vi "PDA_Blast_Acquisition.vi"(4 "Shutter Mode":bool, 5 "Number of Accumulations":i16=5, 6 "error in":errorcluster, 7 "StartIng Mode":T1(ring), 9 "Acquisition Parameters":T2={"Exposure (ms)"=100, "Interval (ms)"=100, "Flush Count"=1, "Trigger"=0} {"Trigger" items=["Disable", "Acquistion", "Cycle"]}) -> (0 "error out":errorcluster, 1 "Pixel Overflow":i32, 2 "PDA Overflow":bool, 3 "Final Data Array":dbl[](array[numeric]) format="%.2f")   [LabVIEW 2019]
doc: "This VI demonstrates acquisition and image display of CCD data\nutilizing the ISA CCD driver.\n\nNote: Specific help is available for each individual control, display and indicator."
uses:
  Globals and TypeDefs/Type Definitions.llb/3 way Status.ctl
  <vilib>/Analysis/baseanly.llb/Mean (DBL).vi
  Globals and TypeDefs/gStatus.vi
  IGA_comm.llb/Controller Version Number.vi
  <vilib>/Analysis/NI_AALBase.lvlib
panel:
  out "Blasttime":u32
  out "Current Mode":T1(ring)
  in  "Tab Control":enum32{"All Accumulations", "Averaged Signal"}(tab)
  out "Display":sgl[][](graph)
  out "Averaged Signal":dbl[](graph)
  out "Avg value":dbl format="%0.2f"
  out "Avg Deviation":dbl format="%0.2f"
  out "Time Used":u32[](array[numeric])
  in  "CCD ADC and Gain":dbl(ring) items=["16 bits Gain 1", "16 bits Gain 2", "16 bits Gain 3", "16 bits Gain 4", "14 bits Gain 1", "14 bits Gain 2"]
  out "Data":u16[][](array[numeric])
  in  "Number of Region":u32=1 min=1 max=1
  # "Total"
  # "Init"
  # "Reset"
  # "SetAcqPara"
  # "SetArea"
  # "Acquisition"
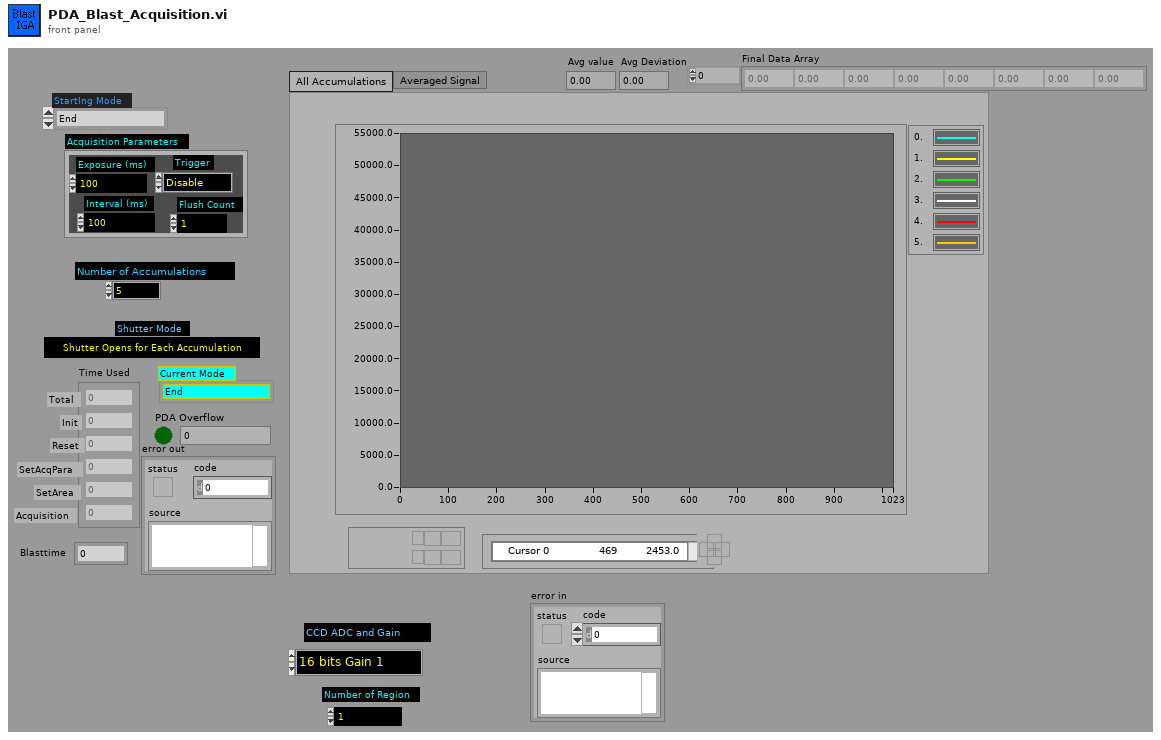
[diagram p1: front panel]
types:
  T1 = enum16{"End", "Init", "Reset", "SetAcqParameter", "SetArea", "AcqData"}
  T2 = cluster{"Exposure (ms)":u32, "Interval (ms)":u32, "Flush Count":i32, "Trigger":u16}
  T3 = typedef "3 way Status.ctl" = u8
  T4 = cluster{"Comm Interface":u16, "BUS":i16, "Address":i16, "Com Port":i32}
  T5 = cluster{"Exposure (ms)":bool, "Interval (ms)":bool, "Flush Count":bool, "Trigger":bool}
  T6 = cluster{"X Origin":u32, "Y Origin":u32, "X Size":u32, "Y Size":u32, "X Bin":u32, "Y Bin":u32}[]
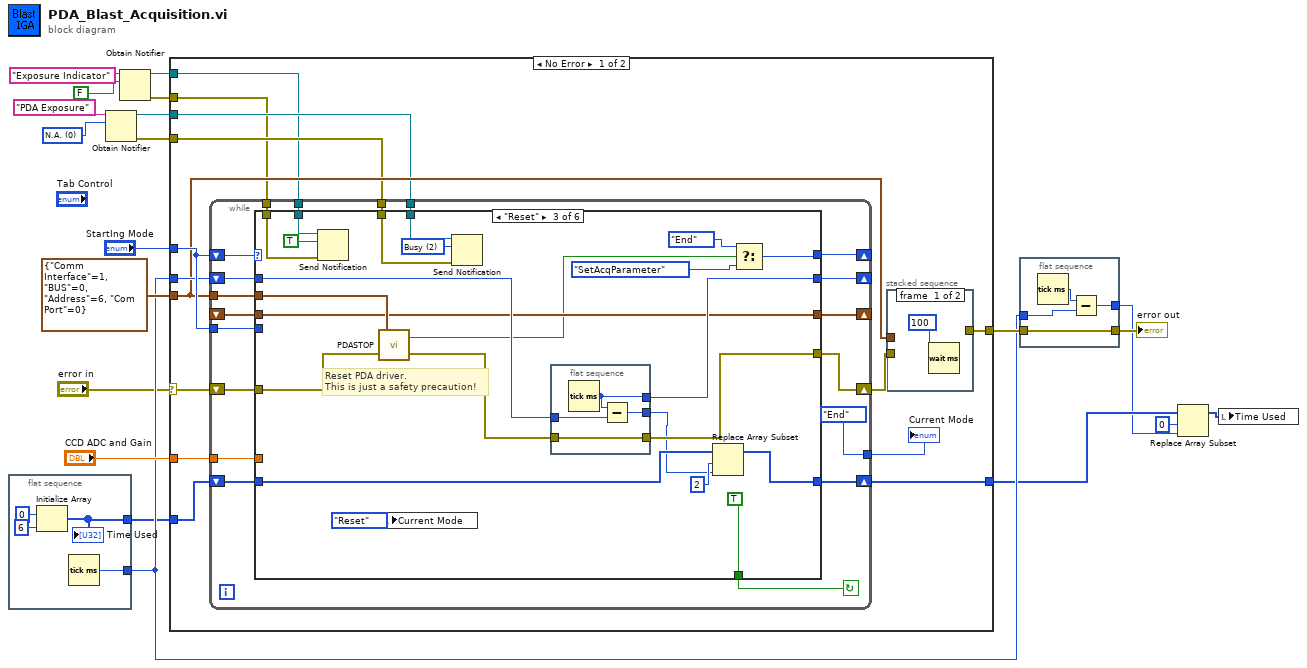
[diagram p0: block diagram]
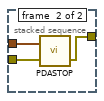
[diagram p2: hidden frame]
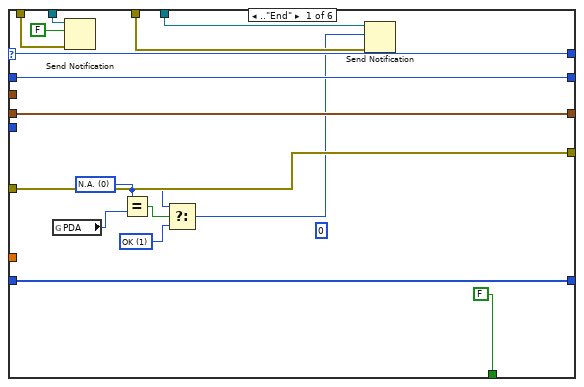
[diagram p3: hidden frame]
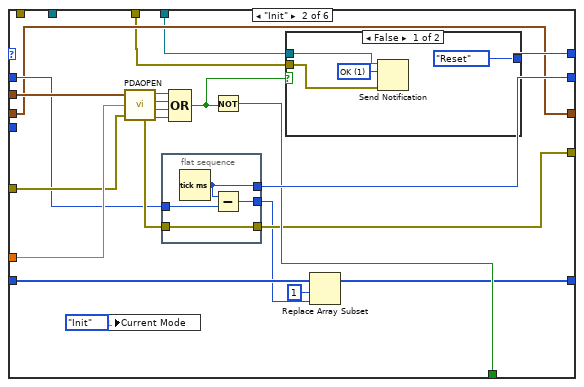
[diagram p4: hidden frame]
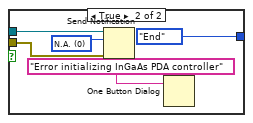
[diagram p5: hidden frame]
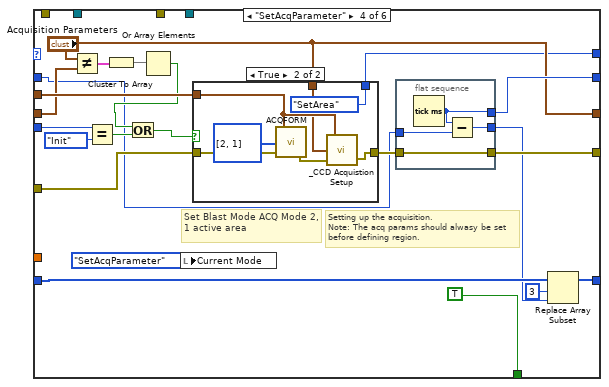
[diagram p6: hidden frame]
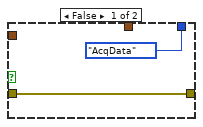
[diagram p7: hidden frame]
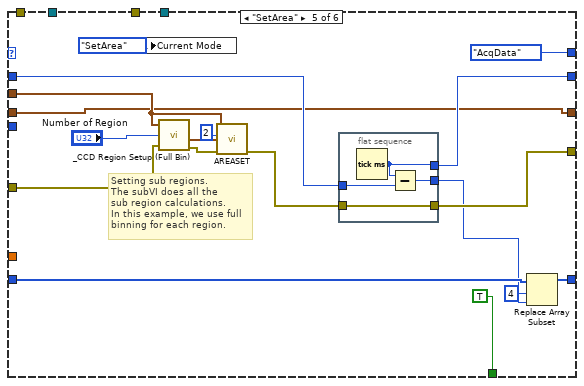
[diagram p8: hidden frame]
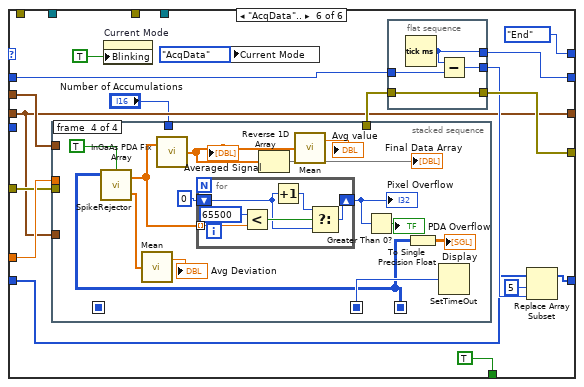
[diagram p9: hidden frame]
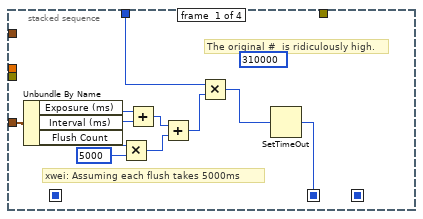
[diagram p10: hidden frame]
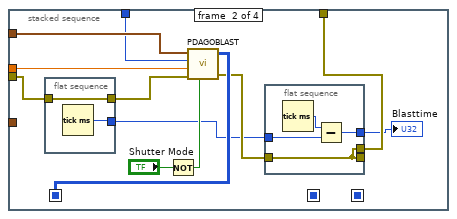
[diagram p11: hidden frame]
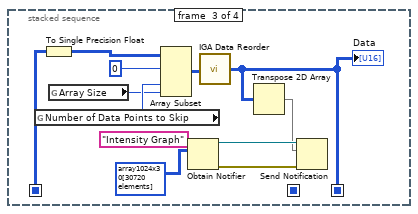
[diagram p12: hidden frame]
diagram:
  w8 = T3 0 items=["N.A.", "OK", "Busy", "Done"] ("Saving")
  n1 = flat-sequence {
    tunnel: [w24] -> w15
    tunnel: [w21] -> w14
    frame #0 {
      n2 = Initialize Array(u32 0 ("element"), 6 ("dimension size")) -> (w21:u32[])
      "Time Used" <- w21
      n3 = Tick Count (ms)() -> (millisecond timer value=w24:u32)
    }
  }
  n4 = Obtain Notifier(name (unnamed)="PDA Exposure", notification data type=w8) -> (notifier out=w7:refnum<notifier>, error out=w6:errorcluster)  [unwired: 2 in, 1 out]
  n5 = Obtain Notifier(name (unnamed)="Exposure Indicator", notification data type=FALSE ("SaveData?")) -> (notifier out=w3:refnum<notifier>, error out=w2:errorcluster)  [unwired: 2 in, 1 out]
  n6 = case shown="No Error" "error in" {
    selector: "error in" -> [w29 w277]
    tunnel: [w38 w277] -> w17
    tunnel: w15 -> [w34 _]
    tunnel: "StartIng Mode" -> [w36 _]
    tunnel: T4 {"Comm Interface"=1, "BUS"=0, "Address"=6, "Com Port"=0} ("Comm Params") -> [w33 _]
    tunnel: "CCD ADC and Gain" -> [w35 _]
    tunnel: w14 -> [w32 w278]
    tunnel: [w31 w278] -> w12
    tunnel: w7 -> [w28 _]
    tunnel: w6 -> [w27 _]
    tunnel: w3 -> [w26 _]
    tunnel: w2 -> [w25 _]
    frame No Error {
      n7 = while {
        tunnel: w35 -> [w57]
        shift-left: _ -> [w58]
        shift-right: [w59] -> _
        shift-left: w36 -> [w51]
        shift-right: [w60] -> _
        shift-right: [w53] -> w37
        shift-left: w29 -> [w56]
        shift-right: [w54] -> _
        shift-left: w34 -> [w55]
        tunnel: w33 -> [w52]
        tunnel: w36 -> [w50]
        shift-right: [w48] -> w31
        shift-left: w32 -> [w49]
        tunnel: [T1."End" ("Current Mode")] -> w30
        tunnel: w28 -> [w46]
        tunnel: w27 -> [w45]
        tunnel: w26 -> [w44]
        tunnel: w25 -> [w43]
        stop <- w61 continue-if-true
        n8 = case shown="\"Reset\"" w51 {
          selector: w51 -> [w76 _ _ _ _ _]
          tunnel: [FALSE w89 TRUE TRUE TRUE TRUE] -> w61
          tunnel: [w76 w86 w121 w145 T1."AcqData" ("InGaAsSS") T1."End" ("InGaAsSS")] -> w60
          tunnel: w58 -> [w75 w85 w128 w155 w182 w199]
          tunnel: [w75 w85 w128 "Acquisition Parameters" w182 w199] -> w59
          tunnel: w57 -> [_ w94 _ _ _ w212]
          tunnel: w56 -> [w73 w93 w134 w160 w176 w211]
          tunnel: w55 -> [w74 w91 w132 w146 w185 w197]
          tunnel: [w74 w90 w131 w157 w186 w208] -> w54
          tunnel: [w73 w88 w130 w158 w187 w209] -> w53
          tunnel: w52 -> [_ w95 w129 w156 w184 w207]
          tunnel: w50 -> [_ _ _ w151 _ _]
          tunnel: w49 -> [w72 w84 w125 w143 w179 w203]
          tunnel: [w72 w81 w126 w142 w180 w202] -> w48
          tunnel: w46 -> [w68 w79 w118 _ _ _]
          tunnel: w45 -> [w67 w78 w117 _ _ _]
          tunnel: w44 -> [w64 _ w115 _ _ _]
          tunnel: w43 -> [w63 _ w114 _ _ _]
          frame .."End" {
            w69 = T3 0 items=["N.A.", "OK", "Busy", "Done"] ("x")
            w65 = T3 1 items=["N.A.", "OK", "Busy", "Done"] ("Saving")
            (unwired) u32 0 ("Read count")
            n9 = global read "gStatus.vi" "PDA"() -> (w71:T3)
            n10 = Send Notification(notification=FALSE, notifier=w64, error in (no error)=w63) -> ()  [unwired: 2 out]
            n11 = Equal?(x=w69, y=w71) -> (x = y?=w70:bool)
            n12 = Select(t=w69, s=w70, f=w65) -> (s? t:f=w66:T3)
            n13 = Send Notification(notification=w66, notifier=w68, error in (no error)=w67) -> ()  [unwired: 2 out]
          }
          frame "Init" {
            n14 = local write "Current Mode"(T1."Init" ("Current Mode")) -> ()
            n15 = call "PDAOPEN.VI"("error in"=w93, "CCD ADC and Gain"=w94, "Comm Params"=w95) -> ("State Error"=w96:bool, "error out"=w92:errorcluster, "Table Error"=w97:bool, "Init Error"=w98:bool, "Boot Error"=w99:bool)  [unwired: 1 out]
            n16 = flat-sequence {
              tunnel: w92 -> [w112]
              tunnel: [w112] -> w88
              tunnel: w91 -> [w111]
              tunnel: [w110] -> w83
              tunnel: [w109] -> w90
              frame #0 {
                n17 = Tick Count (ms)() -> (millisecond timer value=w109:u32)
                n18 = Subtract(x=w109, y=w111) -> (x-y=w110:u32)
              }
            }
            n19 = Compound Arithmetic op=OR(w99, w98, w97, w96) -> (w87:bool)
            n20 = Not(x=w87) -> (.not. x?=w89:bool)
            n21 = case shown="False" w87 {
              tunnel: [T1."Reset" ("InGaAsSS") T1."End" ("InGaAsSS")] -> w86
              tunnel: w79 -> [w102 w106]
              tunnel: w78 -> [w101 w105]
              frame False {
                w100 = T3 1 items=["N.A.", "OK", "Busy", "Done"] ("notification")
                n22 = Send Notification(notification=w100, notifier=w102, error in (no error)=w101) -> ()  [unwired: 2 out]
              }
              frame True {
                w104 = T3 0 items=["N.A.", "OK", "Busy", "Done"] ("notification")
                n23 = Send Notification(notification=w104, notifier=w106, error in (no error)=w105) -> ()  [unwired: 2 out]
                n24 = One Button Dialog(message="Error initializing InGaAs PDA controller") -> ()  [unwired: 1 in, 1 out]
              }
            }
            n25 = Replace Array Subset(array=w84, new element=w83, index=1) -> (w81:u32[])
          }
          frame "Reset" {
            w116 = T3 2 items=["N.A.", "OK", "Busy", "Done"] ("notification")
            # "Reset PDA driver.\nThis is just a safety precaution!"
            n26 = Send Notification(notification=TRUE, notifier=w115, error in (no error)=w114) -> ()  [unwired: 2 out]
            n27 = call "PDASTOP.VI"("error in"=w134, "Comm Params"=w129) -> ("error out"=w133:errorcluster, "Error"=w122:bool)
            n28 = local write "Current Mode"(T1."Reset" ("Current Mode")) -> ()
            n29 = Send Notification(notification=w116, notifier=w118, error in (no error)=w117) -> ()  [unwired: 2 out]
            n30 = flat-sequence {
              tunnel: w133 -> [w139]
              tunnel: [w139] -> w130
              tunnel: w132 -> [w138]
              tunnel: [w137] -> w124
              tunnel: [w136] -> w131
              frame #0 {
                n31 = Tick Count (ms)() -> (millisecond timer value=w136:u32)
                n32 = Subtract(x=w136, y=w138) -> (x-y=w137:u32)
              }
            }
            n33 = Replace Array Subset(array=w125, new element=w124, index=2) -> (w126:u32[])
            n34 = Select(t=T1."End" ("InGaAsSS"), s=w122, f=T1."SetAcqParameter" ("InGaAsSS")) -> (s? t:f=w121:T1)
          }
          frame "SetAcqParameter" {
            # "Setting up the acquisition.\nNote: The acq params should alwasy be set\nbefore defining region."
            # "Set Blast Mode ACQ Mode 2, 1 active area"
            n35 = Not Equal?(x="Acquisition Parameters", y=w155) -> (x != y?=w152:T5)
            n36 = Equal?(x=w151, y=T1."Init") -> (x = y?=w149:bool)
            n37 = Cluster To Array(cluster=w152) -> (array=w153:bool[])
            n38 = Or Array Elements(Boolean array=w153) -> (logical OR=w148:bool)
            n39 = Or(x=w148, y=w149) -> (x .or. y?=w147:bool)
            n40 = local write "Current Mode"(T1."SetAcqParameter" ("Current Mode")) -> ()
            n41 = case shown="True" w147 {
              tunnel: w160 -> [w163 w170]
              tunnel: [w163 w167] -> w159
              tunnel: w156 -> [_ w166]
              tunnel: "Acquisition Parameters" -> [_ w165]
              tunnel: [T1."AcqData" ("InGaAsSS") T1."SetArea" ("InGaAsSS")] -> w145
              frame False {
              }
              frame True {
                n42 = call "ACQFORM.VI"("error in"=w170, "Acquisition Format"=i32[] [2, 1], "Comm Params"=w166) -> ("error out"=w168:errorcluster)  [unwired: 1 out]
                n43 = call "_CCD Acquistion Setup.vi"("error in"=w168, "Acquisition Param"=w165, "Comm Params"=w166) -> ("error out"=w167:errorcluster)  [unwired: 1 out]
              }
            }
            n44 = flat-sequence {
              tunnel: w159 -> [w174]
              tunnel: [w174] -> w158
              tunnel: w146 -> [w173]
              tunnel: [w172] -> w141
              tunnel: [w171] -> w157
              frame #0 {
                n45 = Tick Count (ms)() -> (millisecond timer value=w171:u32)
                n46 = Subtract(x=w171, y=w173) -> (x-y=w172:u32)
              }
            }
            n47 = Replace Array Subset(array=w143, new element=w141, index=3) -> (w142:u32[])
          }
          frame "SetArea" {
            # "Setting sub regions.\nThe subVI does all the\nsub region calculations.\nIn this example, we use full\nbinning for each region."
            n48 = local write "Current Mode"(T1."SetArea" ("Current Mode")) -> ()
            n49 = call "_CCD Region Setup (Full Bin).vi"("Comm Params"=w184, "Number of Regions"="Number of Region", "error in"=w176) -> ("Region Info Array"=w190:T6, "error out"=w175:errorcluster)  [unwired: 2 out]
            n50 = call "AREASET.VI"("error in"=w175, "Region Info Array"=w190, "Acquisition Format"=2, "Comm Params"=w184) -> ("error out"=w188:errorcluster)  [unwired: 3 in, 1 out]
            n51 = flat-sequence {
              tunnel: w188 -> [w196]
              tunnel: [w196] -> w187
              tunnel: w185 -> [w195]
              tunnel: [w194] -> w178
              tunnel: [w193] -> w186
              frame #0 {
                n52 = Tick Count (ms)() -> (millisecond timer value=w193:u32)
                n53 = Subtract(x=w193, y=w195) -> (x-y=w194:u32)
              }
            }
            n54 = Replace Array Subset(array=w179, new element=w178, index=4) -> (w180:u32[])
          }
          frame "AcqData".. {
            n55 = stacked-sequence {
              seq-local: [w228 _ _ _] -> [_ _ _ w270]
              seq-local: [_ w238 _ _] -> [_ _ w254 _]
              seq-local: [_ _ w248 _] -> [_ _ _ w269]
              tunnel: w207 -> [_ w240 _ _]
              tunnel: w212 -> [_ w237 _ _]
              tunnel: w211 -> [_ w235 _ _]
              tunnel: [_ w231 _ _] -> w210
              tunnel: w199 -> [w227 _ _ _]
              tunnel: "Number of Accumulations" -> [w219 w236 _ _]
              frame #0 {
                (unwired) 310000 ("new timeout (10000)")
                # "The original #  is ridiculously high."
                # "xwei: Assuming each flush takes 5000ms"
                n56 = Unbundle By Name(w227) -> ("Exposure (ms)"=w226:u32, "Interval (ms)"=w225:u32, "Flush Count"=w224:i32)
                n57 = Multiply(x=w224, y=5000) -> (x*y=w221:i32)
                n58 = Add(x=w226, y=w225) -> (x+y=w222:u32)
                n59 = Add(x=w222, y=w221) -> (x+y=w220:u32)
                n60 = Multiply(x=w219, y=w220) -> (x*y=w218:u32)
                n61 = SetTimeOut(1:w218) -> (0:w228:i32)
              }
              frame #1 {
                n62 = flat-sequence {
                  tunnel: w235 -> [w246]
                  tunnel: [w246] -> w234
                  tunnel: [w245] -> w230
                  frame #0 {
                    n63 = Tick Count (ms)() -> (millisecond timer value=w245:u32)
                  }
                }
                n64 = Not(x="Shutter Mode") -> (.not. x?=w233:bool)
                n65 = call "PDAGOBLAST.vi"("Comm Params"=w240, "Number of Accumulations"=w236, "CCD ADC and Gain"=w237, "error in"=w234, "Shutter Mode"=w233) -> ("Data"=w238:u16[][], "error out"=w232:errorcluster)  [unwired: 1 out]
                n66 = flat-sequence {
                  tunnel: w232 -> [w241]
                  tunnel: [w241] -> _
                  tunnel: w230 -> [w244]
                  tunnel: [w243] -> w229
                  tunnel: [w241] -> w231
                  frame #0 {
                    n67 = Tick Count (ms)() -> (millisecond timer value=w242:u32)
                    n68 = Subtract(x=w242, y=w244) -> (x-y=w243:u32)
                  }
                }
                "Blasttime" <- w229
              }
              frame #2 {
                n69 = global read "Controller Version Number.vi" "Number of Data Points to Skip"() -> (w257:i8)
                n70 = To Single Precision Float(number=w254) -> ()  [unwired: 1 out]
                n71 = global read "Controller Version Number.vi" "Array Size"() -> (w255:i32)
                n72 = Array Subset(array=w254, index (row)=0 ("Array Index"), index (col)=w257, length (col)=w255) -> (w253:u16[][])  [unwired: 1 in]
                n73 = Obtain Notifier(name (unnamed)="Intensity Graph", notification data type=i32[][] array1024x30[30720 elements] ("Intensity Graph")) -> (notifier out=w250:refnum<notifier>, error out=w249:errorcluster)  [unwired: 2 in, 1 out]
                n74 = call "IGA Data Reorder.VI"("Input Array"=w253) -> ("Output Array"=w248:i32[][])  [unwired: 2 in]
                "Data" <- w248
                n75 = Transpose 2D Array(2D array=w248) -> (transposed array=w247:i32[][])
                n76 = Send Notification(notification=w247, notifier=w250, error in (no error)=w249) -> ()  [unwired: 2 out]
              }
              frame #3 {
                n77 = call "SpikeRejector.vi"("Average Only (T)"=TRUE, "Input Array"=w269) -> ("Sigma Array"=w268:dbl[], "Final Array"=w258:dbl[])  [unwired: 2 in]
                n78 = call-poly <vilib>:"Mean.vi"("X"=w268) -> ("mean"=→"Avg Deviation":dbl)  [unwired: 1 out]
                n79 = call "InGaAs PDA Fix Array.vi"("Input Array"=w258) -> ("Output Array"=w262:dbl[])  [unwired: 2 in]
                "Averaged Signal" <- w262
                n80 = for {
                  tunnel: w258 -> [w276] mode=indexing
                  shift-right: [w271] -> w260
                  shift-left: 0 -> [w272]
                  n81 = Less?(x=65500, y=w276) -> (x < y?=w274:bool)
                  n82 = Increment(x=w272) -> (x+1=w273:i32)
                  n83 = Select(t=w273, s=w274, f=w272) -> (s? t:f=w271:i32)
                }
                "Pixel Overflow" <- w260
                n84 = Reverse 1D Array(array=w262) -> (reversed array=→"Final Data Array":dbl[])
                n85 = call-poly <vilib>:"Mean.vi"("X"=w262) -> ("mean"=→"Avg value":dbl)  [unwired: 1 out]
                n86 = Greater Than 0?(x=w260) -> (x > 0?=→"PDA Overflow":bool)
                n87 = To Single Precision Float(number=w269) -> (single precision float=→"Display":sgl[][])
                n88 = SetTimeOut(1:w270) -> ()  [unwired: 1 out]
              }
            }
            n89 = property on="Current Mode" class="Enum (strict)"("Blinking"=TRUE) -> ()  [unwired: 2 in, 2 out]
            n90 = local write "Current Mode"(T1."AcqData" ("Current Mode")) -> ()
            n91 = flat-sequence {
              tunnel: w210 -> [w217]
              tunnel: [w217] -> w209
              tunnel: w197 -> [w216]
              tunnel: [w215] -> w204
              tunnel: [w214] -> w208
              frame #0 {
                n92 = Tick Count (ms)() -> (millisecond timer value=w214:u32)
                n93 = Subtract(x=w214, y=w216) -> (x-y=w215:u32)
              }
            }
            n94 = Replace Array Subset(array=w203, new element=w204, index=5) -> (w202:u32[])
          }
        }
      }
      "Current Mode" <- w30
      n95 = stacked-sequence {
        tunnel: [_ w42] -> w38
        tunnel: w37 -> [_ w41]
        tunnel: w33 -> [_ w40]
        frame #0 {
          n96 = Wait (ms)(milliseconds to wait=u32 100) -> ()  [unwired: 1 out]
        }
        frame #1 {
          n97 = call "PDASTOP.VI"("error in"=w41, "Comm Params"=w40) -> ("error out"=w42:errorcluster)  [unwired: 1 out]
        }
      }
    }
    frame Error {
    }
  }
  n98 = flat-sequence {
    tunnel: w17 -> [w282]
    tunnel: [w282] -> w16
    tunnel: w15 -> [w281]
    tunnel: [w280] -> w11
    frame #0 {
      n99 = Tick Count (ms)() -> (millisecond timer value=w279:u32)
      n100 = Subtract(x=w279, y=w281) -> (x-y=w280:u32)
    }
  }
  n101 = Replace Array Subset(array=w12, new element=w11, index=0) -> (w10:u32[])
  n102 = local write "Time Used"(w10) -> ()
  "error out" <- w16
